vi "cDAQ - Launch Configuration SW.vi"(8 "error in":errorcluster) -> (0 "error out":errorcluster)   [LabVIEW 2011]
panel:
  out "appended path":path
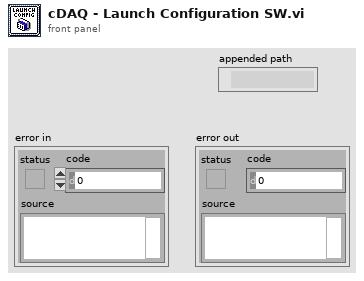
[diagram p1: front panel]
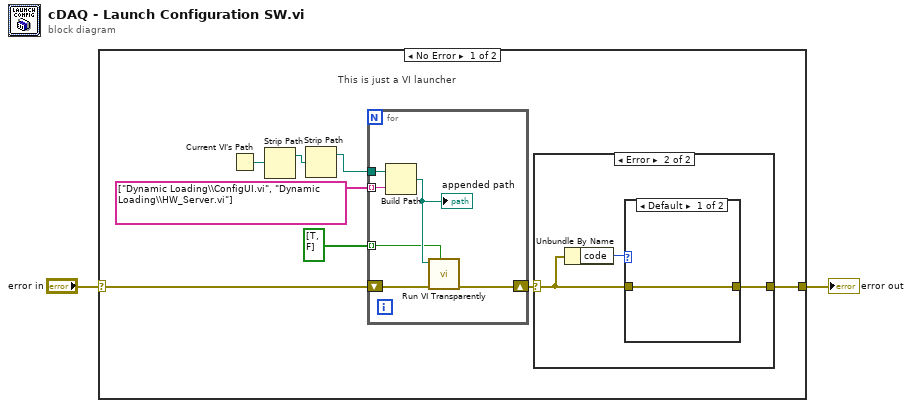
[diagram p0: block diagram]
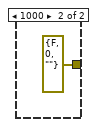
[diagram p3: hidden frame]
diagram:
  n1 = case shown="No Error" "error in" {
    selector: "error in" -> [w3 w23]
    tunnel: [w7 w23] -> w2
    frame No Error {
      # "This is just a VI launcher"
      n2 = Current VI's Path() -> (path=w10:path)
      n3 = Strip Path(path=w10) -> (stripped path=w6:path)  [unwired: 1 out]
      n4 = Strip Path(path=w6) -> (stripped path=w5:path)  [unwired: 1 out]
      n5 = for {
        shift-right: [w21] -> w8
        shift-left: w3 -> [w22]
        tunnel: string[] ["Dynamic Loading\\ConfigUI.vi", "Dynamic Loading\\HW_Server.vi"] -> [w20] mode=indexing
        tunnel: w5 -> [w18]
        tunnel: bool[] [TRUE, FALSE] -> [w17] mode=indexing
        n6 = Build Path(base path=w18, name or relative path=w20) -> (appended path=w19:path)
        "appended path" <- w19
        n7 = call "Run VI Transparently.vi"("Run Transparently? (T)"=w17, "error in"=w22, "vi path"=w19) -> ("error out"=w21:errorcluster)  [unwired: 8 in]
      }
      n8 = case shown="Error" w8 {
        selector: w8 -> [w11 w13]
        tunnel: [w11 w12] -> w7
        frame No Error {
        }
        frame Error {
          n9 = Unbundle By Name(w13) -> ("code"=w14:i32)
          n10 = case shown="Default" w14 {
            tunnel: w13 -> [w15 _]
            tunnel: [w15 errorcluster {"status"=FALSE, "code"=0, "source"=""} ("error IO")] -> w12
            frame Default {
            }
            frame 1000 {
            }
          }
        }
      }
    }
    frame Error {
    }
  }
  "error out" <- w2
